vi "send error info.vi"(8 "error in":errorcluster, 11 "node ref":T1) -> (0 "error cleared":errorcluster, 3 "node ref out":T1)   [LabVIEW 2020, in "Publisher Subscriber.lvlib"]
uses:
  Publisher Subscriber.lvlib
  Controls/node refnum.ctl
  Controls/error info.ctl
  Controls/node dvr data.ctl
  Controls/data cluster.ctl
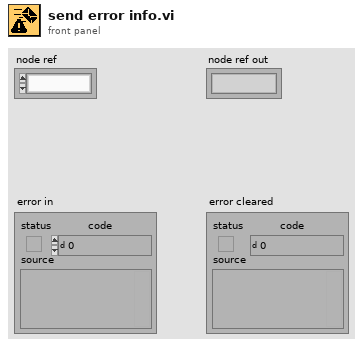
[diagram p1: front panel]
types:
  T1 = typedef "Publisher Subscriber.lvlib/node refnum.ctl" = refnum<k1>
  T2 = typedef "Publisher Subscriber.lvlib/error info.ctl" = cluster{"Module Name":string, "error info":errorcluster}
  T3 = typedef "Publisher Subscriber.lvlib/node dvr data.ctl" = cluster{"queue ref":refnum<queue>, "subscription map ref":refnum<data-value>, "Command":string, "Data":variant, "Subscriptions []":set{string}, "variable dvr refs":refnum<data-value>}
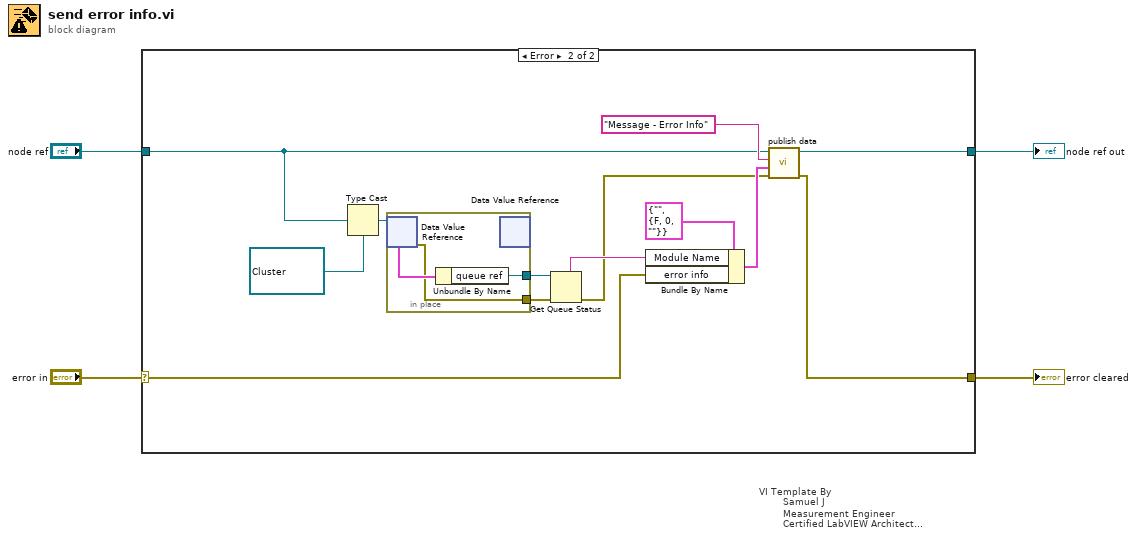
[diagram p0: block diagram]
diagram:
  n1 = case "VI Template By\n        Samuel J\n        Measurement Engineer\n        Certified LabVIEW Architect\n        Vestas Technology R&D Chennai" shown="Error" "error in" {
    selector: "error in" -> [w6 w15]
    tunnel: [w6 w14] -> w3
    tunnel: "node ref" -> [w5 w10]
    tunnel: [w5 w19] -> w1
    frame No Error {
    }
    frame Error {
      n2 = Type Cast(type=refnum<data-value> refnum ("data value reference"), x=w10) -> (*(type *) &x=w13:refnum<data-value>)
      n3 = in-place {
        in-place-border: [w21] -> w12
        in-place-border: [w20] -> w11
        n4 = in-place-dvr #1(w13) -> (w22:T3, w20:errorcluster)
        n5 = Unbundle By Name(w22) -> ("queue ref"=w21:refnum<queue>)
        n6 = in-place-dvr #1() -> ()  [unwired: 1 in, 2 out]
      }
      n7 = Get Queue Status(queue=w12, error in (no error)=w11) -> (queue name=w9:string, error out=w8:errorcluster)  [unwired: 1 in, 6 out]
      n8 = Bundle By Name(cluster=T2 {"Module Name"="", "error info"={"status"=FALSE, "code"=0, "source"=""}} ("error info"), "Module Name"=w9, "error info"=w15) -> (w16:T2)
      n9 = call "publish data.vi"("error in"=w8, "data in"=w16, "command"="Message - Error Info", "refnum in"=w10) -> ("error out"=w14:errorcluster, "refnum out"=w19:T1)  [unwired: 6 in]
    }
  }
  "error cleared" <- w3
  "node ref out" <- w1
